vi "COBS_Test.vi"() -> ()   [LabVIEW 2015, in "Shore Library.lvlib"]
uses:
  Shore Library.lvlib
  <userlib>/_OpenG.lib/numeric/numeric.llb/Random Number Within Range - DBL__ogtk.vi
panel:
  out "x-y":u32
  out "Original 2":u8[](array[numeric])
  out "Stuffed 2":u8[](array[numeric])
  out "Unstuffed 2":u8[](array[numeric])
  out "logical AND 2":bool
  out "logical AND":bool
  out "logical And":bool
  out "Unstuffed":u8[](array[numeric])
  out "Stuffed":u8[](array[numeric])
  out "Original":u8[](array[numeric])
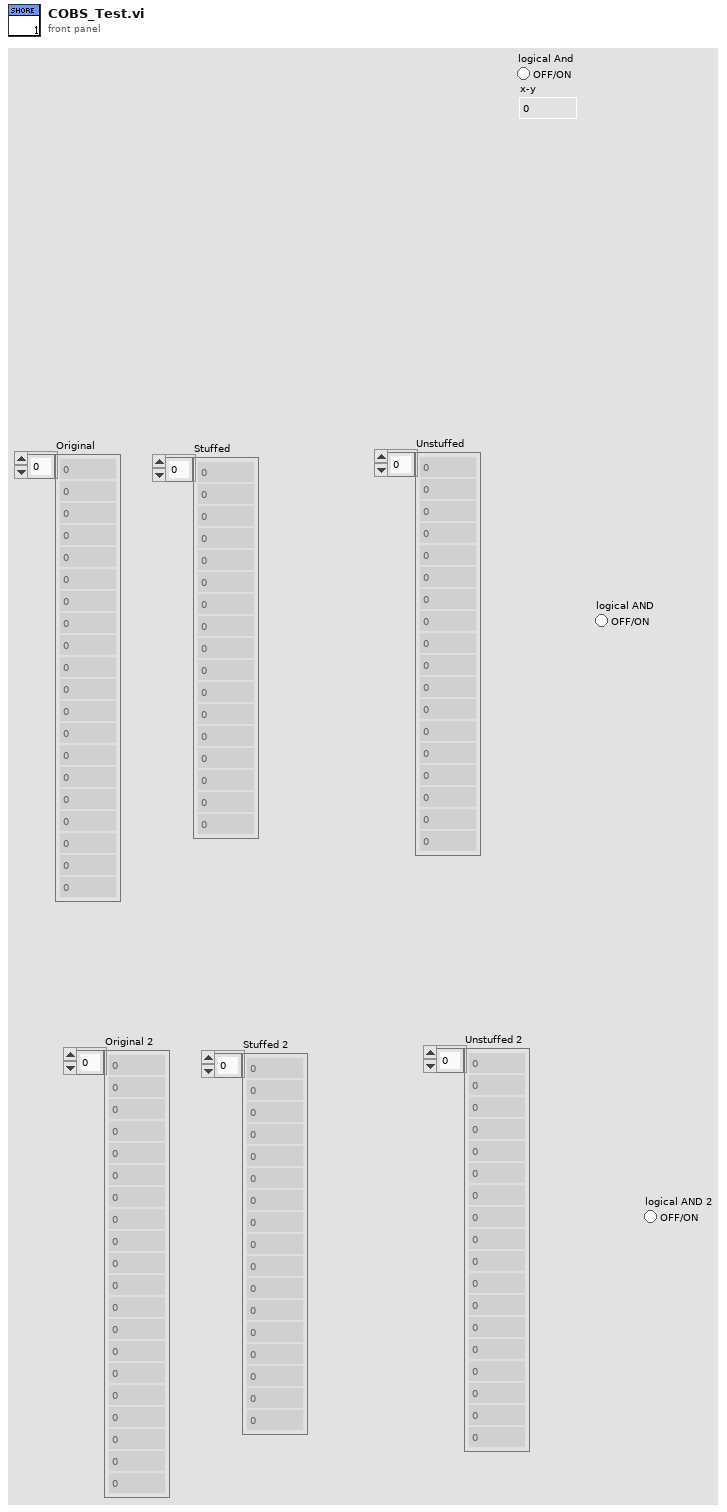
[diagram p1: front panel]
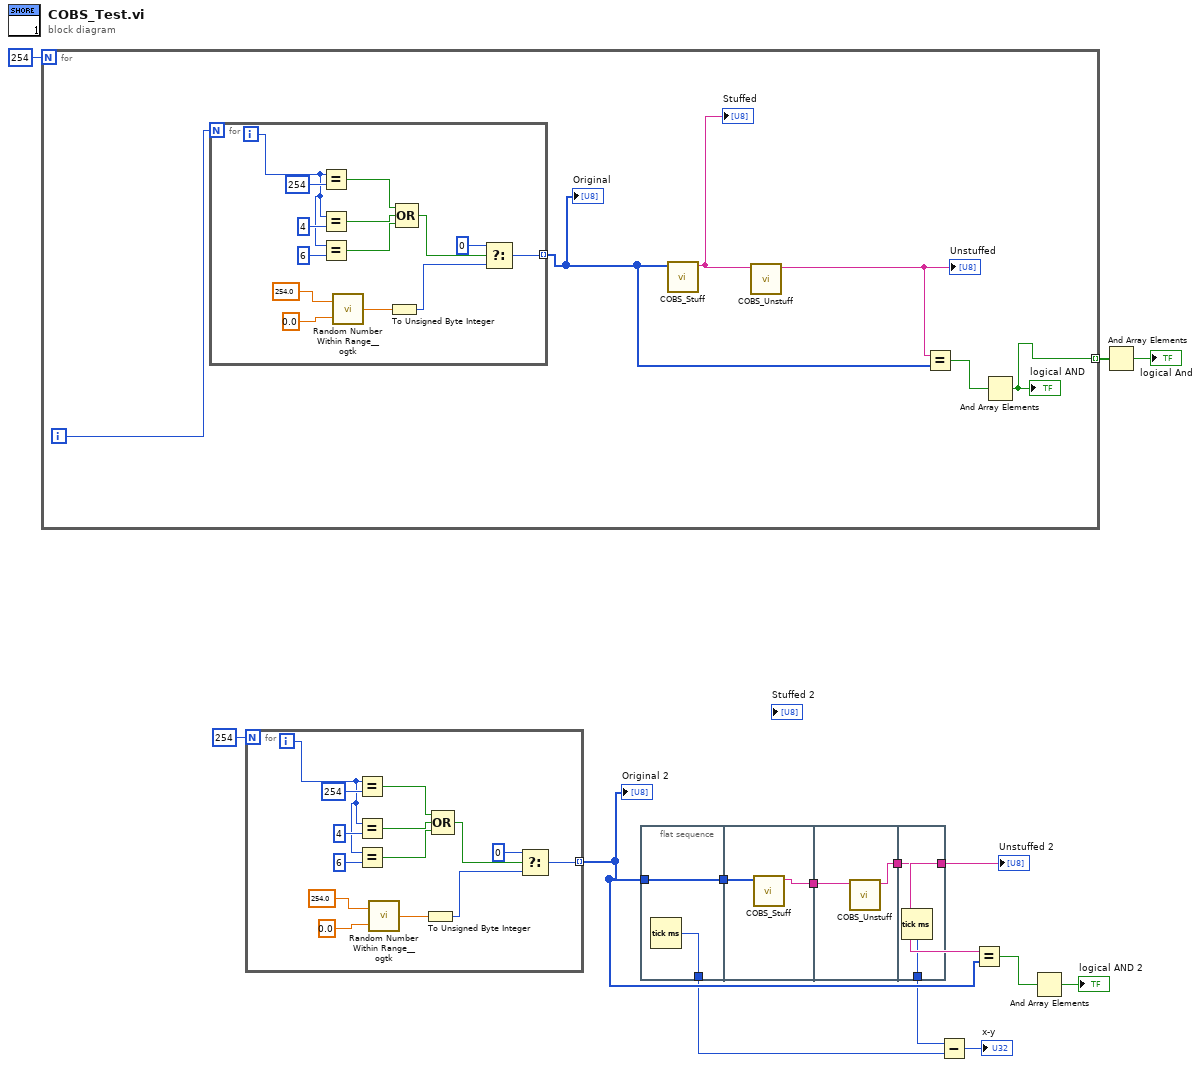
[diagram p0: block diagram]
diagram:
  n1 = for {
    N: 254 -> [_]
    tunnel: [w16] -> w12 mode=indexing
    i -> [w15]
    n2 = for {
      N: w15 -> [_]
      tunnel: [w31] -> w18 mode=indexing
      i -> [w23]
      n3 = Equal?(x=w23, y=254) -> (x = y?=w29:bool)
      n4 = Equal?(x=w23, y=4) -> (x = y?=w28:bool)
      n5 = Equal?(x=w23, y=6) -> (x = y?=w27:bool)
      n6 = call-poly <userlib>:"Random Number Within Range__ogtk.vi"("High"=254.0, "Low"=0.0 ("High")) -> ("Random Number"=w32:dbl)  [unwired: 3 in]
      n7 = To Unsigned Byte Integer(number=w32) -> (unsigned 8bit integer=w22:u8)
      n8 = Compound Arithmetic op=OR(w29, w28, w27) -> (w24:bool)
      n9 = Select(t=u8 0, s=w24, f=w22) -> (s? t:f=w31:u8)
    }
    "Original" <- w18
    n10 = call "COBS_Stuff.vi"("Raw data"=w18) -> ("Stuffed Data"=w19:string)  [unwired: 9 in, 1 out]
    "Stuffed" <- w19
    n11 = call "COBS_Unstuff.vi"("Suffed data"=w19) -> ("Unstuffed String"=w20:string)  [unwired: 8 in, 2 out]
    "Unstuffed" <- w20
    n12 = Equal?(x=w20, y=w18) -> (x = y?=w17:bool)
    n13 = And Array Elements(Boolean array=w17) -> (logical AND=w16:bool)
    "logical AND" <- w16
  }
  n14 = for {
    N: 254 -> [_]
    tunnel: [w45] -> w6 mode=indexing
    i -> [w37]
    n15 = Equal?(x=w37, y=254) -> (x = y?=w43:bool)
    n16 = Equal?(x=w37, y=4) -> (x = y?=w42:bool)
    n17 = Equal?(x=w37, y=6) -> (x = y?=w41:bool)
    n18 = call-poly <userlib>:"Random Number Within Range__ogtk.vi"("High"=254.0, "Low"=0.0 ("High")) -> ("Random Number"=w46:dbl)  [unwired: 3 in]
    n19 = To Unsigned Byte Integer(number=w46) -> (unsigned 8bit integer=w36:u8)
    n20 = Compound Arithmetic op=OR(w43, w42, w41) -> (w38:bool)
    n21 = Select(t=u8 0, s=w38, f=w36) -> (s? t:f=w45:u8)
  }
  "Original 2" <- w6
  n22 = flat-sequence {
    tunnel: w6 -> [w50]
    tunnel: [w50] -> w5
    tunnel: [w49] -> w2
    tunnel: [w51] -> w8
    tunnel: w5 -> [w52]
    tunnel: w8 -> [w54]
    tunnel: [w53] -> w4
    tunnel: [w56] -> w7
    tunnel: w4 -> [w56]
    tunnel: [w55] -> w3
    frame #0 {
      n23 = Tick Count (ms)() -> (millisecond timer value=w49:u32)
    }
    frame #1 {
      n24 = call "COBS_Stuff.vi"("Raw data"=w52) -> ("Stuffed Data"=w51:string)  [unwired: 9 in, 1 out]
    }
    frame #2 {
      n25 = call "COBS_Unstuff.vi"("Suffed data"=w54) -> ("Unstuffed String"=w53:string)  [unwired: 8 in, 2 out]
    }
    frame #3 {
      n26 = Tick Count (ms)() -> (millisecond timer value=w55:u32)
    }
  }
  n27 = Subtract(x=w3, y=w2) -> (x-y=→"x-y":u32)
  n28 = Equal?(x=w7, y=w6) -> (x = y?=w10:bool)
  n29 = And Array Elements(Boolean array=w10) -> (logical AND=→"logical AND 2":bool)
  n30 = And Array Elements(Boolean array=w12) -> (logical AND=→"logical And":bool)
  "Unstuffed 2" <- w7
